vi "Player Info.vi"(11 "Rain in":refnum<class "Rain.lvclass">) -> (1 "Victory Speech":string, 2 "Name":string, 3 "Rain out":refnum<class "Rain.lvclass">)   [LabVIEW 2015, in "Rain.lvclass"]
uses:
  Rain.lvclass
  Square/Square.lvclass
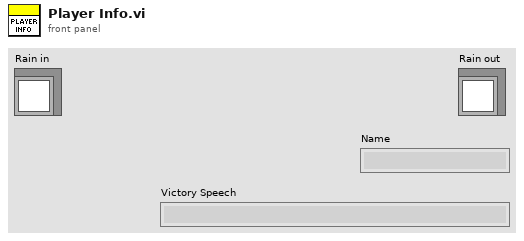
[diagram p1: front panel]
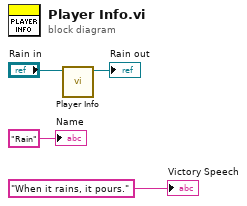
[diagram p0: block diagram]
diagram:
  n1 = call-parent "Player Info.vi"("Square in"="Rain in") -> ("Square out"=→"Rain out":refnum<class "Rain.lvclass">)  [unwired: 8 in, 2 out]
  "Name" <- "Rain"
  "Victory Speech" <- "When it rains, it pours."
